vi "WFM MNGR Get RF Waveform.vi"(8 "error in (no error)":errorcluster, 10 "Waveform to Retrieve":string, 11 "WFM MNGR in":refnum<class "QPA MSMT Waveform Manager.lvclass">) -> (0 "error out":errorcluster, 2 "RF Waveform":T1, 3 "WFM MNGR out":refnum<class "QPA MSMT Waveform Manager.lvclass">)   [LabVIEW 2016, in "QPA MSMT Waveform Manager.lvclass"]
uses:
  QPA MSMT Waveform Manager.lvclass
  Controls/RF Waveform.ctl
  QPA MSMT Waveform Manager.lvclass/QPA MSMT Waveform Manager.ctl
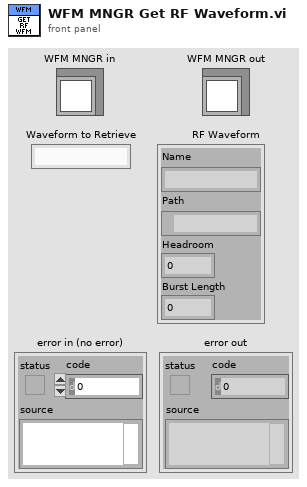
[diagram p1: front panel]
types:
  T1 = typedef "QPA MSMT Waveform Manager.lvclass/RF Waveform.ctl" = cluster{"Name":string, "Path":path, "Headroom":dbl, "Burst Length":dbl}
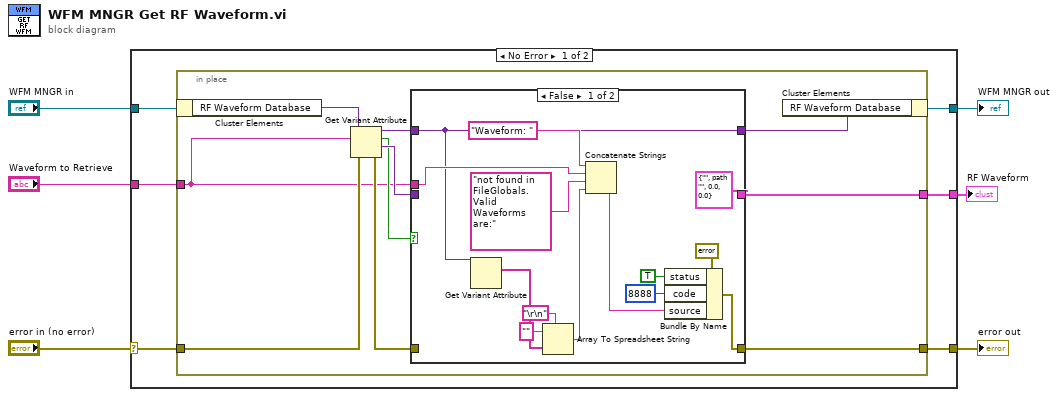
[diagram p0: block diagram]
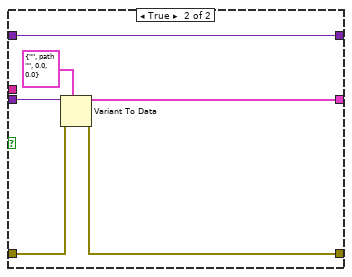
[diagram p2: hidden frame]
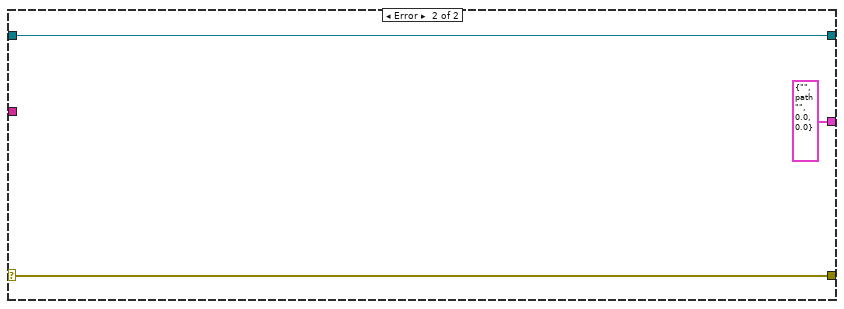
[diagram p3: hidden frame]
diagram:
  n1 = case shown="No Error" "error in (no error)" {
    selector: "error in (no error)" -> [w10 w45]
    tunnel: [w9 w45] -> w5
    tunnel: [w11 w44] -> w3
    tunnel: "WFM MNGR in" -> [w12 w44]
    tunnel: "Waveform to Retrieve" -> [w8 _]
    tunnel: [w7 T1 {"Name"="", "Path"=path "", "Headroom"=0.0, "Burst Length"=0.0} ("RF Waveform")] -> w1
    frame No Error {
      n2 = in-place {
        in-place-border: w10 -> [w21]
        in-place-border: [w18] -> w9
        in-place-border: w8 -> [w15]
        in-place-border: [w17] -> w7
        n3 = in-place-cluster #1(w12) -> ("RF Waveform Database"=w22:variant)
        n4 = Get Variant Attribute(Variant=w22, name=w15, error in=w21) -> (duplicate Variant=w14:variant, found=w16:bool, value=w20:variant, error out=w19:errorcluster)  [unwired: 1 in]
        n5 = case shown="False" w16 {
          tunnel: w20 -> [_ w42]
          tunnel: w19 -> [_ w41]
          tunnel: [w24 w40] -> w18
          tunnel: [T1 {"Name"="", "Path"=path "", "Headroom"=0.0, "Burst Length"=0.0} ("RF Waveform") w38] -> w17
          tunnel: w15 -> [w26 _]
          tunnel: w14 -> [w23 w37]
          tunnel: [w23 w37] -> w13
          frame False {
            n6 = Get Variant Attribute(Variant=w23) -> (names=w31:string[])  [unwired: 3 in, 3 out]
            n7 = Array To Spreadsheet String(delimiter (Tab)="\r\n", array=w31, 3:"" ("format string")) -> (spreadsheet string=w29:string)
            n8 = Concatenate Strings("Waveform: " ("source"), w26, "not found in FileGlobals.  Valid Waveforms are:" ("string"), w29) -> (w28:string)
            n9 = Bundle By Name(cluster=errorcluster {"status"=FALSE, "code"=0, "source"=""} ("error out"), "status"=TRUE, "code"=8888, "source"=w28) -> (w24:errorcluster)
          }
          frame True {
            n10 = Variant To Data(error in=w41, type=T1 {"Name"="", "Path"=path "", "Headroom"=0.0, "Burst Length"=0.0} ("RF Waveform"), Variant=w42) -> (data=w38:T1, error out=w40:errorcluster)
          }
        }
        n11 = in-place-cluster #1("RF Waveform Database"=w13) -> (w11:refnum<class "QPA MSMT Waveform Manager.lvclass">)
      }
    }
    frame Error {
    }
  }
  "error out" <- w5
  "WFM MNGR out" <- w3
  "RF Waveform" <- w1
